vi "subsetupRxHWParameters.vi"(0 "IVI Refnum in":refnum<k15>, 5 "Rx Parameters":T1, 11 "error in (no error)":errorcluster) -> (4 "IVI Refnum out":refnum<k15>, 6 "Rx Parameters":T1, 15 "error out":errorcluster)   [LabVIEW 2017]
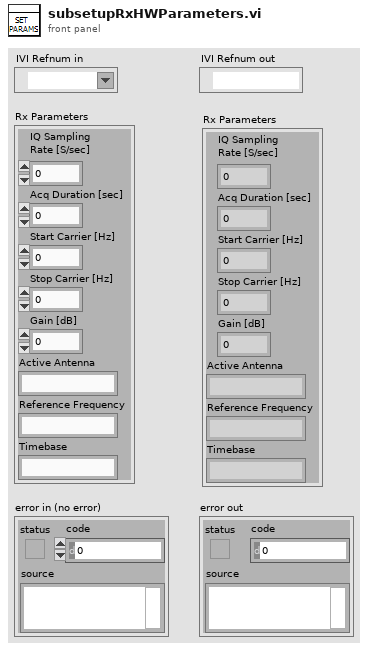
[diagram p1: front panel]
types:
  T1 = cluster{"IQ Sampling\nRate [S/sec]":dbl, "Acq Duration [sec]":dbl, "Start Carrier [Hz]":dbl, "Stop Carrier [Hz]":dbl, "Gain [dB]":dbl, "Active Antenna":string, "Reference Frequency":string, "Timebase":string}
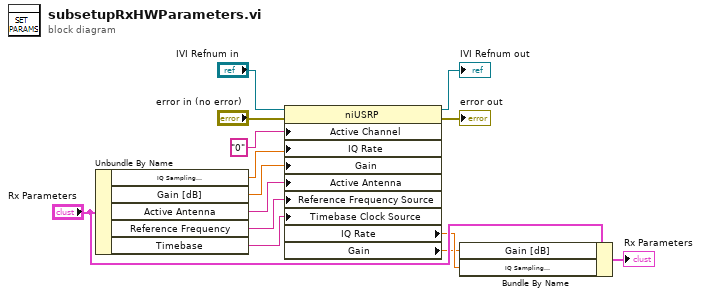
[diagram p0: block diagram]
diagram:
  n1 = Unbundle By Name("Rx Parameters") -> ("IQ Sampling\nRate [S/sec]"=w5:dbl, "Gain [dB]"=w6:dbl, "Active Antenna"=w7:string, "Reference Frequency"=w8:string, "Timebase"=w9:string)
  n2 = property class="niUSRP"(reference="IVI Refnum in", error in="error in (no error)", "Active Channel"="0", "IQ Rate"=w5, "Gain"=w6, "Active Antenna"=w7, "Reference Frequency Source"=w8, "Timebase Clock Source"=w9) -> (reference out=→"IVI Refnum out":refnum<k15>, error out=→"error out":errorcluster, "IQ Rate"=w3:dbl, "Gain"=w1:dbl)
  n3 = Bundle By Name(cluster="Rx Parameters", "Gain [dB]"=w1, "IQ Sampling\nRate [S/sec]"=w3) -> (→"Rx Parameters":T1)
